vi "matlabscript.vi"(7 "base de temps":i32, 8 "error in (no error)":errorcluster, 9 "Table Control":string[][](array[string]), 10 "show system state":i32, 11 "solver data":string) -> (0 "error out":errorcluster)   [LabVIEW 2019]
panel:
  out "concatenated string":string
  out "données plantes":string
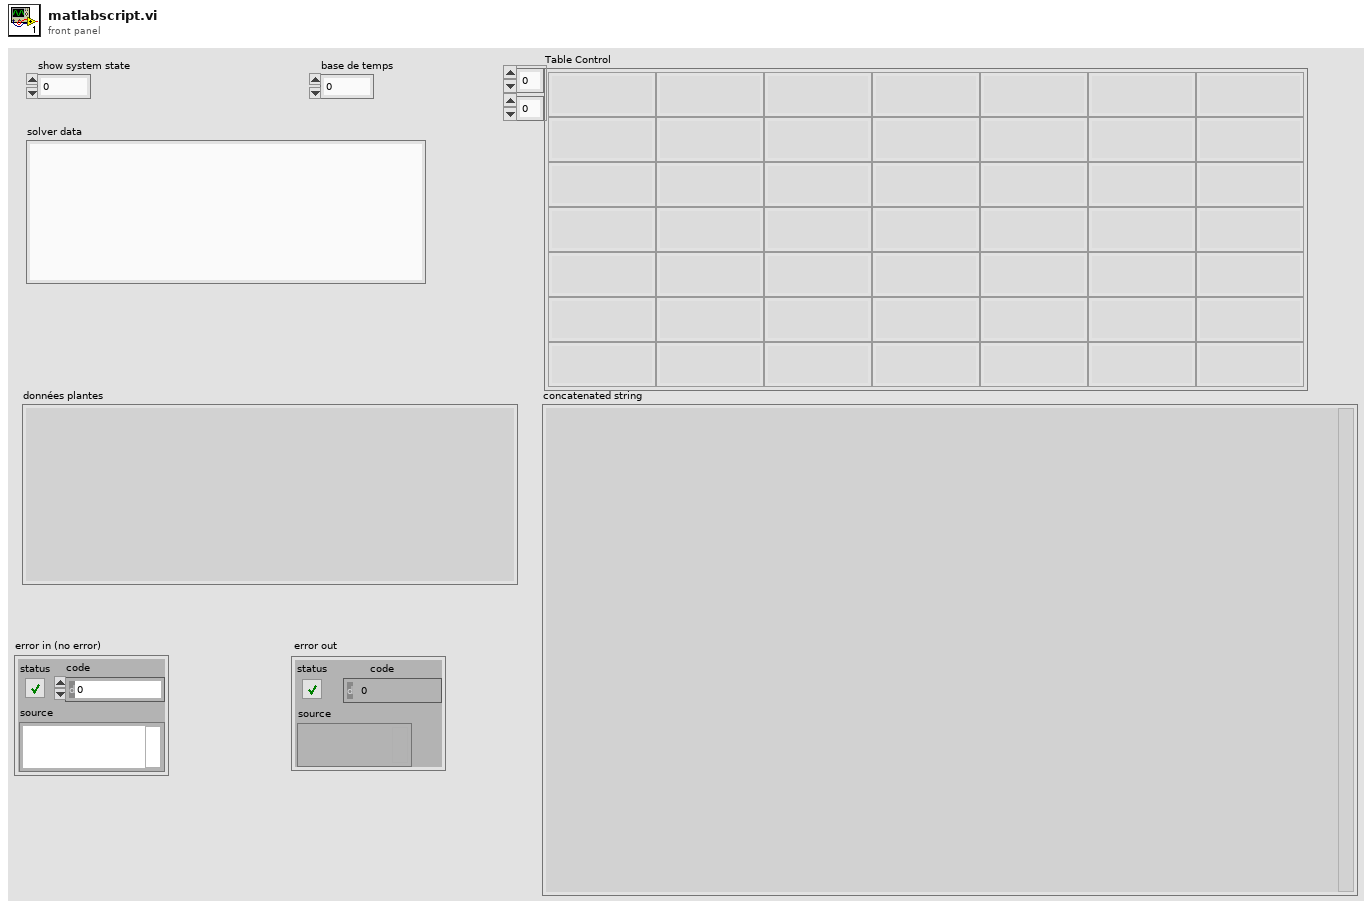
[diagram p1: front panel]
types:
  T1 = enum16{"open", "replace", "create", "open or create", "replace or create", "replace or create with confirmation"}
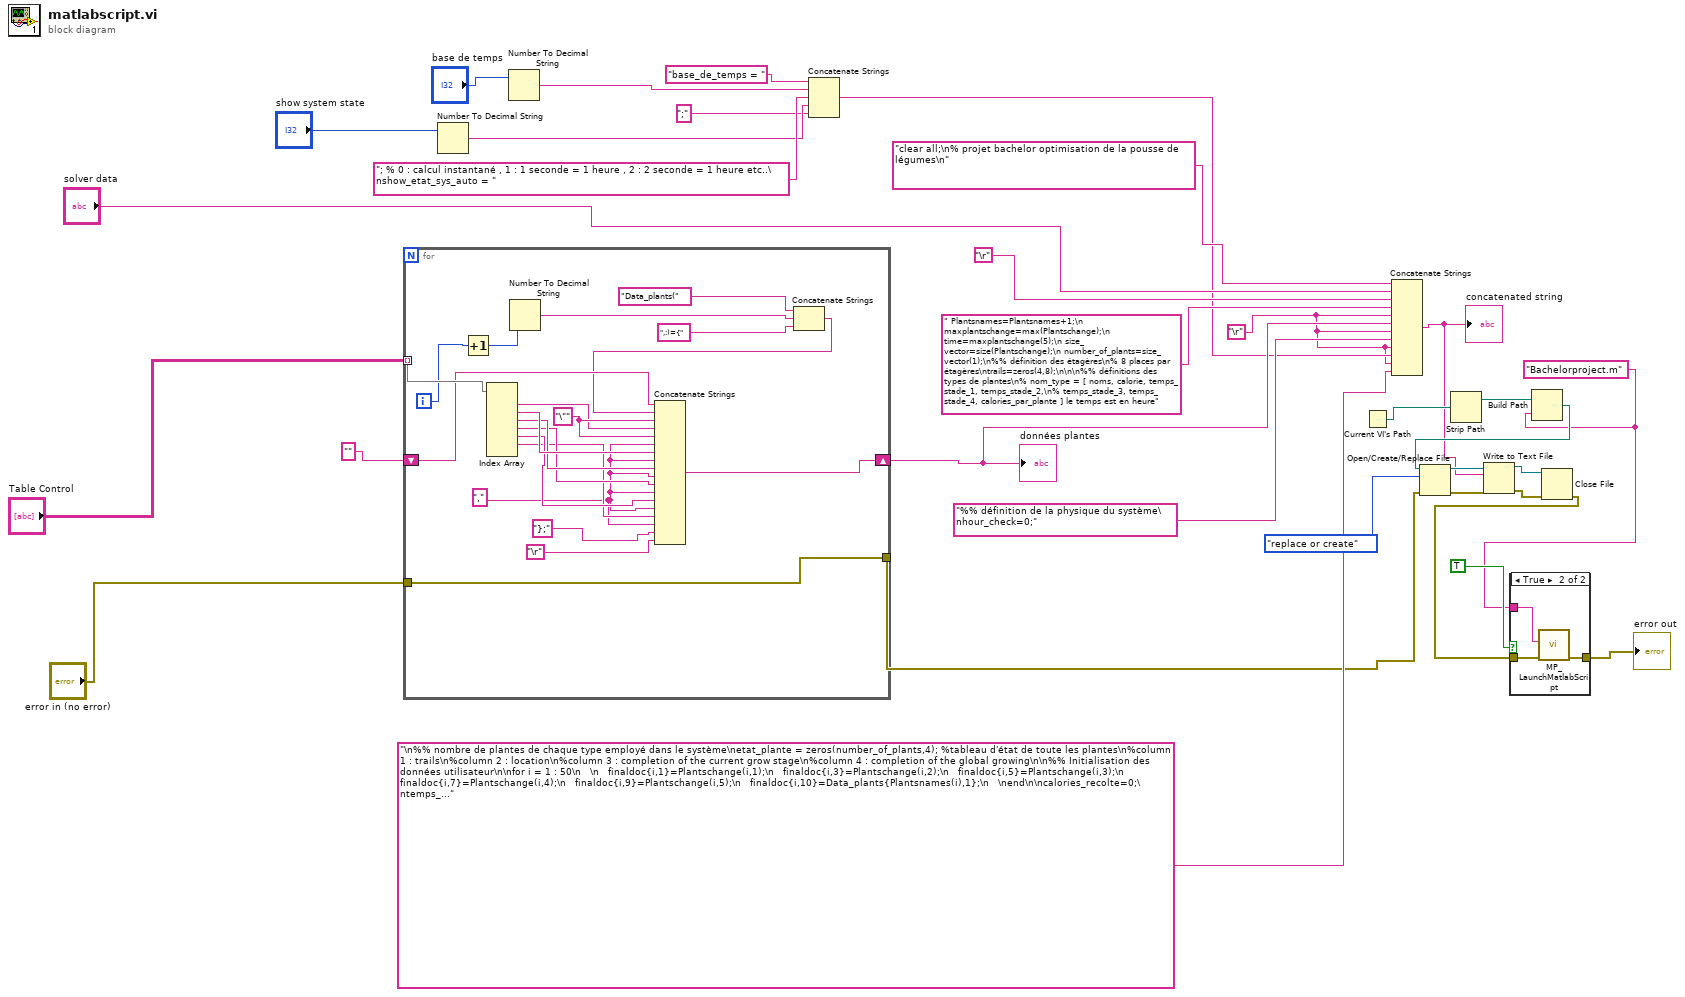
[diagram p0: block diagram]
diagram:
  w1 = "Bachelorproject.m"
  w16 = "\r"
  n1 = for {
    tunnel: "Table Control" -> [w53] mode=indexing
    shift-right: [w52] -> w26
    shift-left: "" -> [w51]
    tunnel: "error in (no error)" -> [w34]
    tunnel: [w34] -> w5
    i -> [w50]
    w44 = "\""
    w37 = ","
    n2 = Increment(x=w50) -> (x+1=w49:i32)
    n3 = Index Array(array=w53) -> (element #1=w43:string, element #2=w42:string, element #3=w41:string, element #4=w40:string, element #5=w39:string, element #6=w38:string)  [unwired: 7 in, 1 out]
    n4 = Number To Decimal String(number=w49) -> (decimal integer string=w48:string)  [unwired: 1 in]
    n5 = Concatenate Strings("Data_plants(", w48, ",:)={") -> (w45:string)
    n6 = Concatenate Strings(w51, w45, w44, w43, w44, w37, w42, w37, w41, w37, w40, w37, w39, w37, w38, w37, "};", "\r") -> (w52:string)
  }
  "données plantes" <- w26
  n7 = Number To Decimal String(number="show system state") -> (decimal integer string=w19:string)  [unwired: 1 in]
  n8 = Number To Decimal String(number="base de temps") -> (decimal integer string=w21:string)  [unwired: 1 in]
  n9 = Concatenate Strings("base_de_temps = ", w21, "; % 0 : calcul instantané , 1 : 1 seconde = 1 heure , 2 : 2 seconde = 1 heure etc..\nshow_etat_sys_auto = ", w19, ";") -> (w17:string)
  n10 = Current VI's Path() -> (path=w10:path)
  n11 = Concatenate Strings("clear all;\n% projet bachelor optimisation de la pousse de légumes\n", "solver data", "\r", " Plantsnames=Plantsnames+1;\n maxplantschange=max(Plantschange);\n time=maxplantschange(5);\n size_vector=size(Plantschange);\n number_of_plants=size_vector(1);\n%% définition des étagères\n% 8 places par étagères\ntrails=zeros(4,8);\n\n\n%% définitions des types de plantes\n% nom_type = [ noms, calorie, temps_stade_1, temps_stade_2,\n% temps_stade_3, temps_stade_4, calories_par_plante ] le temps est en heure", w16, w26, w16, "%% définition de la physique du système\nhour_check=0;", w16, w17, w16, "\n%% nombre de plantes de chaque type employé dans le système\netat_plante = zeros(number_of_plants,4); %tableau d'état de toute les plantes\n%column 1 : trails\n%column 2 : location\n%column 3 : completion of the current grow stage\n%column 4 : completion of the global growing\n\n%% Initialisation des données utilisateur\n\nfor i = 1 : 50\n   \n   finaldoc{i,1}=Plantschange(i,1);\n   finaldoc{i,3}=Plantschange(i,2);\n   finaldoc{i,5}=Plantschange(i,3);\n   finaldoc{i,7}=Plantschange(i,4);\n   finaldoc{i,9}=Plantschange(i,5);\n   finaldoc{i,10}=Data_plants{Plantsnames(i),1};\n   \nend\n\ncalories_recolte=0;\ntemps_ecoule=0;\ncompteur=1;\n%% bloucle du programme\nwhile (temps_ecoule<time+1)\nt1=fix(clock);\n%récolte\n\n\n\n    i=1;\n    while i<number_of_plants+1\n          if(temps_ecoule==Plantschange(i,5))\n            calories_recolte=calories_recolte+Data_plants{Plantsnames(i),2};\n            trails(4,etat_plante(i,2))=0; \n            etat_plante(i,1)=-1;\n            etat_plante(i,2)=-1;\n            etat_plante(i,3)=100;\n            etat_plante(i,4)=100;\n           \n          end\n        i=i+1;\n    end\n\n%etagere 4\n\ni=1;\nwhile i<number_of_plants+1\n        if(temps_ecoule==Plantschange(i,4))\n            i_etagere=1;\n            while i_etagere<9\n                if trails(4,i_etagere)== 0\n                   trails(3,etat_plante(i,2))=0;\n                   trails(4,i_etagere)= 1;\n                   etat_plante(i,1)=4;\n                   etat_plante(i,2)=i_etagere;\n                   finaldoc{i,8}=i_etagere;\n                   i_etagere=9;\n                end\n                i_etagere=i_etagere+1;\n            end\n        end\n        i=i+1;\nend\n\n%etagere 3\n\n\ni=1;\nwhile i<number_of_plants+1\n        if(temps_ecoule==Plantschange(i,3))\n            i_etagere=1;\n            while i_etagere<9\n                if trails(3,i_etagere)== 0\n                   trails(2,etat_plante(i,2))=0;\n                   trails(3,i_etagere)= 1;\n                   etat_plante(i,1)=3;\n                   etat_plante(i,2)=i_etagere;\n                   finaldoc{i,6}=i_etagere;\n                   i_etagere=9;\n                end\n                i_etagere=i_etagere+1;\n            end\n        end\n        i=i+1;\nend\n\n%etagere 2\n\ni=1;\nwhile i<number_of_plants+1    \n        if(temps_ecoule==Plantschange(i,2))\n            i_etagere=1;\n            while i_etagere<9\n                if trails(2,i_etagere)== 0\n                   trails(1,etat_plante(i,2))=0;\n                   trails(2,i_etagere)= 1;\n                   etat_plante(i,1)=2;\n                   etat_plante(i,2)=i_etagere;\n                   finaldoc{i,4}=i_etagere;\n                   i_etagere=9;\n                end\n                i_etagere=i_etagere+1;\n            end\n        end\n     i=i+1;\nend\n\n%etagere 1\n\ni=1;                                        %\nwhile i<number_of_plants+1                    %\n     if (temps_ecoule==Plantschange(i,1))           \n          i_etagere=1;\n          while i_etagere<9\n              if trails(1,i_etagere)== 0\n                   trails(1,i_etagere)= 1;\n                   etat_plante(i,1)=1;\n                   etat_plante(i,2)=i_etagere;\n                   finaldoc{i,2}=i_etagere;\n                  i_etagere=9;\n              end\n              i_etagere=i_etagere+1;\n          end\n     end\n      i=i+1;\nend\n\n\n\n\n\n\n\n\n\n    \n%mise à jour de la valeur de croissance\ni=1;\nwhile i<number_of_plants+1\n    if (Plantschange(i,1)<temps_ecoule) && (Plantschange(i,5)>temps_ecoule)\n        etat_plante(i,4)=((temps_ecoule-Plantschange(i,1))/(Plantschange(i,5)-Plantschange(i,1))*100);\n        etat_plante(i,3)=((temps_ecoule-Plantschange(i,etat_plante(i,1)))/(Plantschange(i,etat_plante(i,1)+1)-Plantschange(i,etat_plante(i,1)))*100);\n    end\n\ni=i+1;\nend\n\nif (mod(temps_ecoule,show_etat_sys_auto)==0) && (show_etat_sys_auto~=0)\n for i=1:50\n     for i2=1:4\n     summary{i,i2}=etat_plante(i,i2);\n     end\n     summary{i,5}=Data_plants{Plantsnames(i),1};\n end\n cal=sprintf(\"calories récoltés : %d\",calories_recolte);\n summary{51,1}=cal;\n filename=sprintf(\"summar_hour_ %d .txt\",temps_ecoule);\n writecell(summary,filename)\nend\n\nif (base_de_temps ~= 0)\nwhile (hour_check==0)\n    t2=fix(clock);\n    time_elapsed=etime(t2,t1);\n    if time_elapsed>base_de_temps\n        hour_check=1;\n    end\nend\nend\nhour_check=0;    \ntemps_ecoule=temps_ecoule+1;\nend\n\n writecell(finaldoc,\"finaldoc.txt\");") -> (w6:string)
  "concatenated string" <- w6
  n12 = Strip Path(path=w10) -> (stripped path=w9:path)  [unwired: 1 out]
  n13 = Build Path(base path=w9, name or relative path=w1) -> (appended path=w8:path)
  n14 = Open/Create/Replace File(file path (use dialog)=w8, error in=w5, operation (0:open)=T1."replace or create") -> (refnum out=w12:refnum<file>, error out=w4:errorcluster)  [unwired: 3 in, 1 out]
  n15 = Write to Text File(file (use dialog)=w12, text=w6, error in=w4) -> (refnum out=w11:refnum<file>, error out=w3:errorcluster)  [unwired: 1 in, 1 out]
  n16 = Close File(refnum=w11, error in=w3) -> (error out=w2:errorcluster)  [unwired: 1 out]
  n17 = case shown="True" TRUE {
    tunnel: w2 -> [w54 w57]
    tunnel: [w54 w56] -> w14
    tunnel: w1 -> [_ w55]
    frame False {
    }
    frame True {
      n18 = call "MP_LaunchMatlabScript.vi"("error in (no error)"=w57, "matlab script name with extension"=w55) -> ("error out"=w56:errorcluster)  [unwired: 5 in, 4 out]
    }
  }
  "error out" <- w14
